vi "GetText.vi"(8 "error in":errorcluster, 11 "bin datalogger editor node in":refnum<class "Binary datalogger editor node.lvclass">) -> (0 "error out":errorcluster, 1 "additional text":string, 2 "text":string, 3 "bin datalogger editor node out":refnum<class "Binary datalogger editor node.lvclass">, 4 "glyph":string)   [LabVIEW 2013, in "Binary datalogger editor node.lvclass"]
uses:
  Binary datalogger editor node.lvclass
  <vilib>/NI/Tag Bus Data Framework/Configuration Editor/Classes/Module editor node/module editor node.lvclass
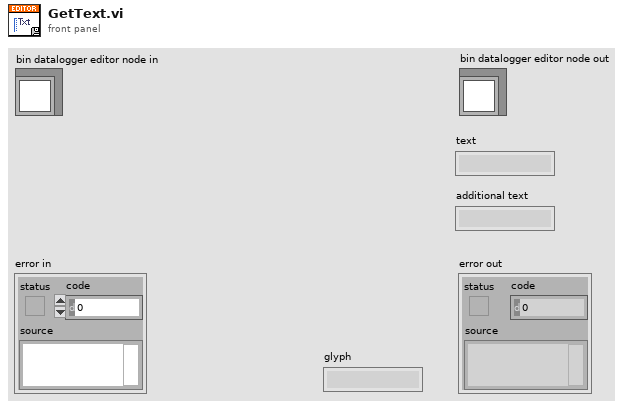
[diagram p1: front panel]
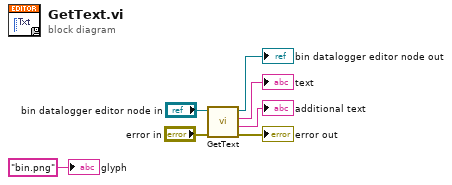
[diagram p0: block diagram]
diagram:
  n1 = call-parent "GetText.vi"("error in"="error in", "Module Editor Node in"="bin datalogger editor node in") -> ("error out"=→"error out":errorcluster, "additional text"=→"additional text":string, "text"=→"text":string, "Module Editor Node out"=→"bin datalogger editor node out":refnum<class "Binary datalogger editor node.lvclass">)  [unwired: 5 in, 1 out]
  "glyph" <- "bin.png" ("glyph")
